vi "ScreenshotSingleVIs.vi"(6 "Title Prefix In":string, 8 "error in":errorcluster, 9 "Picture Save Location":path, 11 "VI Path 1":path) -> (0 "error out":errorcluster)   [LabVIEW 2015]
uses:
  Utilities/Arguments.ctl
  Screenshots/VI Screenshots.ctl
  Screenshots/Screenshot Info.ctl
  Screenshots/Screenshot Type.ctl
  Utilities/FilePaths.ctl
  Utilities/VIDiff_Utilities.lvlib
  Screenshots/VIDiff_Screenshots.lvlib
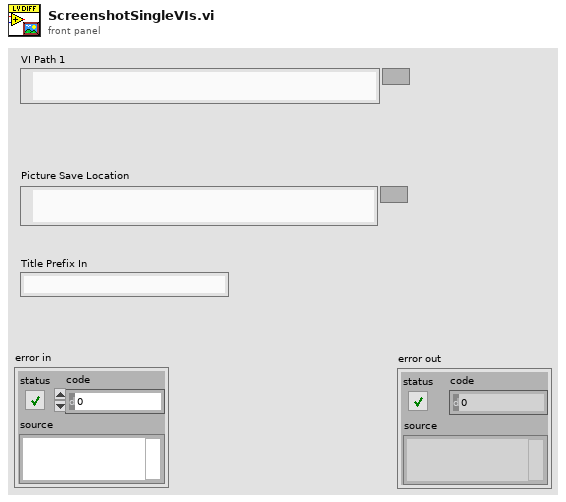
[diagram p1: front panel]
types:
  T1 = typedef "VIDiff_Screenshots.lvlib/Screenshot Type.ctl" = enum16{"Unknown", "Front Panel", "Connector Pane", "Block Diagram", "VI Hierarchy"}
  T2 = typedef "VIDiff_Screenshots.lvlib/VI Screenshots.ctl" = cluster{"Front Panel Screenshots":T3[], "Block Diagram Screenshots":T3[], "Connector Pane Screenshots":T3[], "VI Hierarchy Screenshots":T3[], "Unknown Screenshots":T3[], "vi reference":refnum<vi>, "File Paths":cluster{"File Path":path, "Container Path":path}, "Name":string}
  T3 = typedef "VIDiff_Screenshots.lvlib/Screenshot Info.ctl" = cluster{"Screenshot Path":path, "Screenshot Type":T1, "VI Paths":T4}
  T4 = typedef "VIDiff_Utilities.lvlib/FilePaths.ctl" = cluster{"File Path":path, "Container Path":path}
  T5 = typedef "VIDiff_Utilities.lvlib/Arguments.ctl" = cluster{"VI 1 Path":path, "VI 2 Path":path, "Picture Save Location":path, "Screenshot Title":string}
  T6 = typedef "VIDiff_Utilities.lvlib/Output Folders.ctl" = cluster{"combined":path, "vi1shots":path, "vi2shots":path, "Picture Save Location":path}
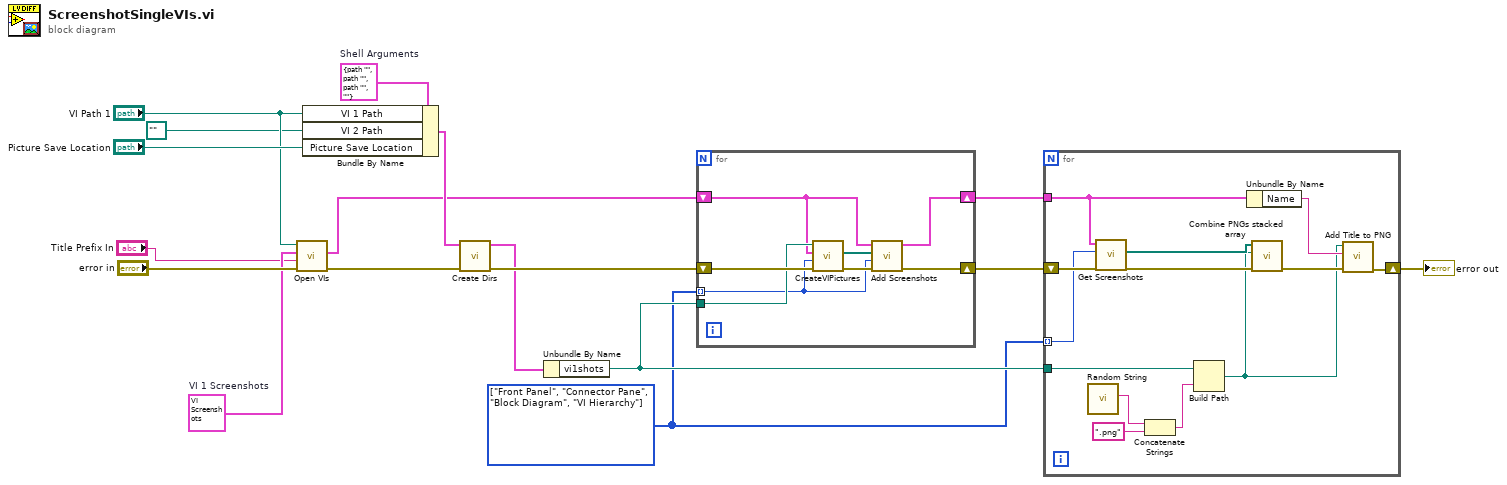
[diagram p0: block diagram]
diagram:
  w2 = T1[] [enum."Front Panel", enum."Connector Pane", enum."Block Diagram", enum."VI Hierarchy"] items=["Unknown", "Front Panel", "Connector Pane", "Block Diagram", "VI Hierarchy"]
  w13 = T2 {"Front Panel Screenshots"=[], "Block Diagram Screenshots"=[], "Connector Pane Screenshots"=[], "VI Hierarchy Screenshots"=[], "Unknown Screenshots"=[], "vi reference"=refnum, "File Paths"={"File Path"=path "", "Container Path"=path ""}, "Name"=""}  # VI 1 Screenshots
  w17 = T5 {"VI 1 Path"=path "", "VI 2 Path"=path "", "Picture Save Location"=path "", "Screenshot Title"=""}  # Shell Arguments
  n1 = call "Open VIs.vi"("error in (no error)"="error in", "Title Prefix In"="Title Prefix In", "VI Screenshots"=w13, "VI Path"="VI Path 1") -> ("error out"=w6:errorcluster, "VI Screenshots out"=w12:T2)  [unwired: 6 in]
  n2 = Bundle By Name(cluster=w17, "VI 1 Path"="VI Path 1", "VI 2 Path"=path "" ("VI Path 2"), "Picture Save Location"="Picture Save Location") -> (w14:T5)
  n3 = call "Create Dirs.vi"("error in (no error)"=w6, "Shell Arguments"=w14) -> ("error out"=w11:errorcluster, "Output Folders"=w10:T6)  [unwired: 8 in]
  n4 = Unbundle By Name(w10) -> ("vi1shots"=w4:path)
  n5 = for {
    tunnel: w2 -> [w19] mode=indexing
    shift-right: [w18] -> w3
    shift-left: w11 -> [w25]
    tunnel: w4 -> [w24]
    shift-right: [w22] -> w5
    shift-left: w12 -> [w21]
    n6 = call "CreateVIPictures.vi"("error in (no error)"=w25, "Capture Target"=w19, "VI 1 Screenshots"=w21, "Picture Save Location"=w24) -> ("error out"=w20:errorcluster, "Screenshot Files"=w23:path[])  [unwired: 6 in]
    n7 = call "Add Screenshots.vi"("error in (no error)"=w20, "Screenshot Type"=w19, "Screenshot Paths"=w23, "VI Screenshots In"=w21) -> ("error out"=w18:errorcluster, "VI Screenshots Out"=w22:T2)  [unwired: 6 in]
  }
  n8 = for {
    tunnel: w5 -> [w29]
    tunnel: w4 -> [w35]
    tunnel: w2 -> [w33] mode=indexing
    shift-right: [w26] -> w1
    shift-left: w3 -> [w34]
    n9 = call "Random String.vi"() -> ("Random String"=w38:string)  [unwired: 11 in]
    n10 = call "Get Screenshots.vi"("error in (no error)"=w34, "Screenshot Type"=w33, "VI Screenshots In"=w29) -> ("error out"=w31:errorcluster, "Screenshot Paths"=w32:path[])  [unwired: 7 in]
    n11 = Concatenate Strings(w38, ".png" ("string")) -> (w36:string)
    n12 = Build Path(base path=w35, name or relative path=w36) -> (appended path=w27:path)
    n13 = Unbundle By Name(w29) -> ("Name"=w28:string)
    n14 = call "Combine PNGs stacked array.vi"("error in (no error)"=w31, "Output File"=w27, "Input Files"=w32) -> ("error out"=w30:errorcluster)  [unwired: 8 in]
    n15 = call "Add Title to PNG.vi"("error in (no error)"=w30, "Title String"=w28, "PNG File"=w27) -> ("error out"=w26:errorcluster)  [unwired: 8 in]
  }
  "error out" <- w1
